vi "Configure Measure Layer Trigger Source.vi"(5 "Enable Auto Measure Delay (F: Disable)":bool, 6 "Measure Timer Interval (0.1)":dbl=0.1 format="%#.6g", 7 "Measure Delay (0 s)":dbl format="%#.6g", 8 "error in (no error)":errorcluster, 9 "Measure Count (1)":i32=1, 10 "Measure Source (1: Immediate)":i32(ring)=1 items=["Hold"=0, "Immediate"=1, "Manual"=3, "Bus"=4, "Trigger Link"=5, "External Triggering"=6, "Timer "=7], 11 "VISA resource name":refnum<visa-resource-name>) -> (0 "error out":errorcluster, 3 "VISA resource name out":refnum<visa-resource-name>)   [LabVIEW 2016, in "Keithley 6517.lvlib"]
doc: "Configures the source, count, delay and time interval for the Measure Layer (Trigger) of the trigger model. \n\n<B>Note:</B>\n(1)<B>Models 6517A, 6517B:</B> The trigger model consists of 3 layers, the Arm Layer, the Scan Layer (Arm2), and the Measure Layer (Trigger).\n(2)<B>Model 6514:</B> The trigger model consists of 2 layers: Arm Layer & Measure Layer (Trigger)."
uses:
  <instrlib>/Keithley 6517/Keithley 6517.lvlib
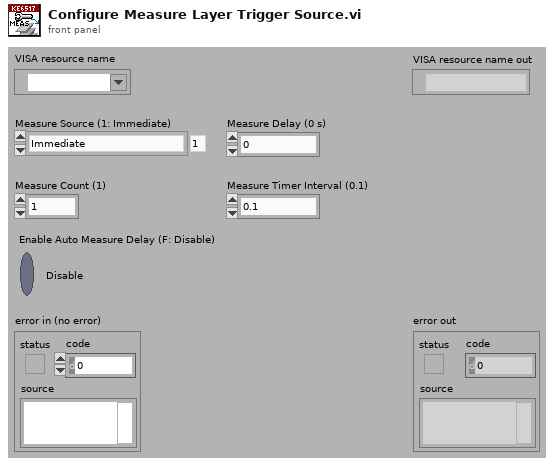
[diagram p1: front panel]
types:
  T1 = typedef "Keithley 6517.lvlib/Extended User Data.ctl" = cluster{"Instrument Model":i32}
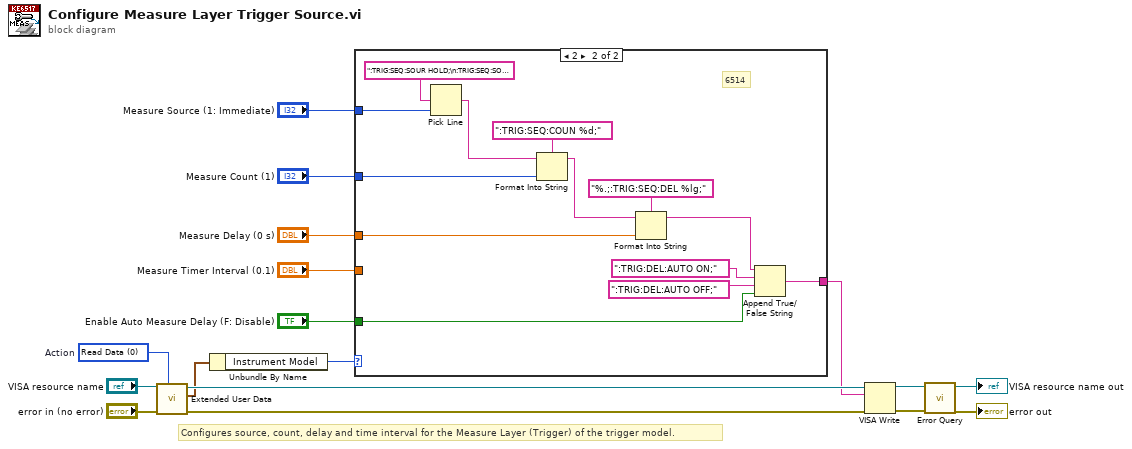
[diagram p0: block diagram]
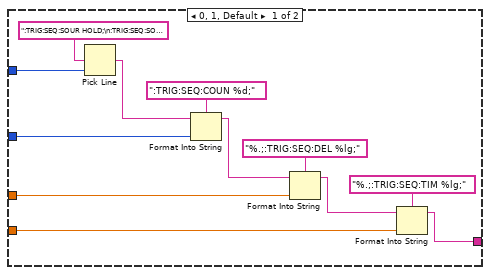
[diagram p2: hidden frame]
diagram:
  w3 = u16 0 items=["Read Data", "Write Data", "Clear Data", "Clear ALL Data"]  # Action
  # "Configures source, count, delay and time interval for the Measure Layer (Trigger) of the trigger model."
  n1 = call <instrlib>:"Extended User Data.vi"("Action (0: Read Data)"=w3, "error in (no error)"="error in (no error)", "VISA resource name"="VISA resource name") -> ("error out"=w7:errorcluster, "User Data Out"=w5:T1, "VISA resource name out"=w6:refnum<visa-resource-name>)  [unwired: 6 in]
  n2 = Unbundle By Name(w5) -> ("Instrument Model"=w4:i32)
  n3 = case shown="2" w4 {
    tunnel: "Measure Count (1)" -> [w28 w41]
    tunnel: "Measure Delay (0 s)" -> [w25 w38]
    tunnel: "Measure Timer Interval (0.1)" -> [w23 _]
    tunnel: "Measure Source (1: Immediate)" -> [w21 w36]
    tunnel: "Enable Auto Measure Delay (F: Disable)" -> [_ w31]
    tunnel: [w18 w30] -> w1
    frame 0, 1, Default {
      n4 = Pick Line(multi-line string=":TRIG:SEQ:SOUR HOLD;\n:TRIG:SEQ:SOUR IMM;\n\n:TRIG:SEQ:SOUR MAN;\n:TRIG:SEQ:SOUR BUS;\n:TRIG:SEQ:SOUR TLIN;\n:TRIG:SEQ:SOUR EXT;\n:TRIG:SEQ:SOUR TIM;", line index=w21) -> (output string=w20:string)  [unwired: 1 in]
      n5 = Format Into String(format string=":TRIG:SEQ:COUN %d;", initial string=w20, w28) -> (resulting string=w27:string)  [unwired: 1 in, 1 out]
      n6 = Format Into String(format string="%.;:TRIG:SEQ:DEL %lg;", initial string=w27, w25) -> (resulting string=w19:string)  [unwired: 1 in, 1 out]
      n7 = Format Into String(format string="%.;:TRIG:SEQ:TIM %lg;", initial string=w19, w23) -> (resulting string=w18:string)  [unwired: 1 in, 1 out]
    }
    frame 2 {
      # "6514"
      n8 = Pick Line(multi-line string=":TRIG:SEQ:SOUR HOLD;\n:TRIG:SEQ:SOUR IMM;\n\n:TRIG:SEQ:SOUR MAN;\n:TRIG:SEQ:SOUR BUS;\n:TRIG:SEQ:SOUR TLIN;\n:TRIG:SEQ:SOUR EXT;\n:TRIG:SEQ:SOUR TIM;", line index=w36) -> (output string=w35:string)  [unwired: 1 in]
      n9 = Format Into String(format string=":TRIG:SEQ:COUN %d;", initial string=w35, w41) -> (resulting string=w40:string)  [unwired: 1 in, 1 out]
      n10 = Format Into String(format string="%.;:TRIG:SEQ:DEL %lg;", initial string=w40, w38) -> (resulting string=w34:string)  [unwired: 1 in, 1 out]
      n11 = Append True/False String(1:w31, 2:":TRIG:DEL:AUTO OFF;", 3:":TRIG:DEL:AUTO ON;", 4:w34) -> (0:w30:string)
    }
  }
  n12 = VISA Write(VISA resource name=w6, write buffer=w1, error in (no error)=w7) -> (VISA resource name out=w14:refnum<visa-resource-name>, error out=w13:errorcluster)  [unwired: 1 out]
  n13 = call <instrlib>:"Error Query.vi"("error in (no error)"=w13, "VISA resource name"=w14) -> ("error out"=→"error out":errorcluster, "VISA resource name out"=→"VISA resource name out":refnum<visa-resource-name>)  [unwired: 6 in, 2 out]
